vi "DatalogFile.vi"() -> ()   [LabVIEW 2019]
panel:
  in  "Boolean 2":bool
  out "Boolean":bool=TRUE
  in  "Write File":bool
  in  "Numeric 4":dbl
  in  "Numeric 3":dbl
  in  "Numeric 2":dbl
  in  "Numeric":dbl
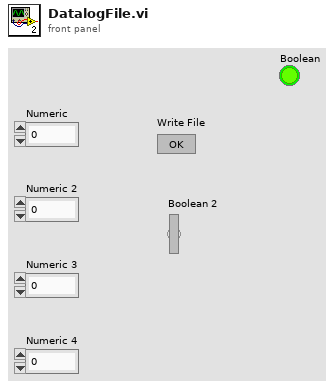
[diagram p1: front panel]
types:
  T1 = enum16{"open", "replace", "create", "open or create", "replace or create", "replace or create with confirmation"}
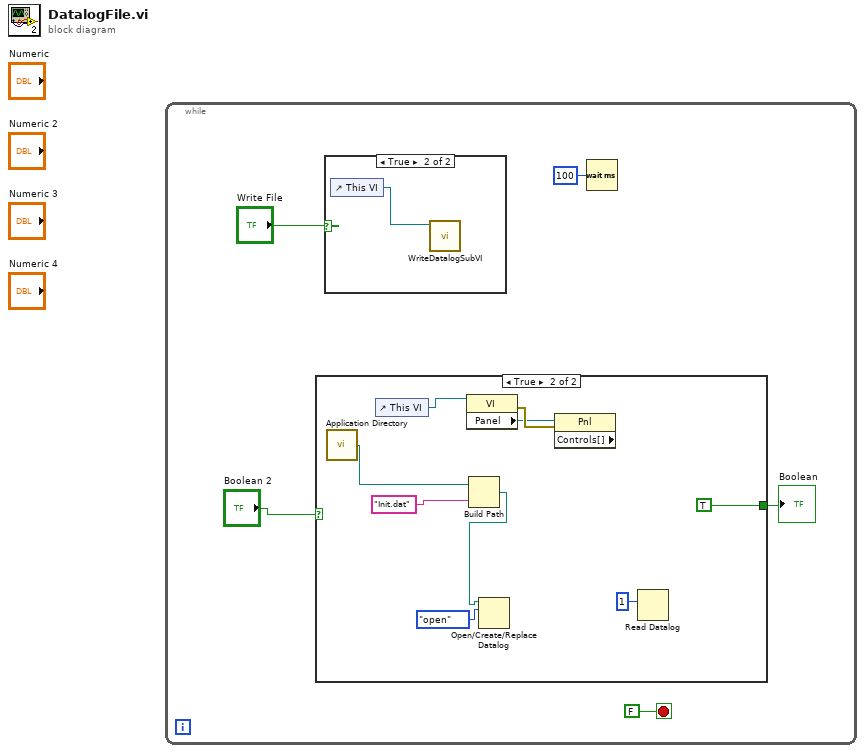
[diagram p0: block diagram]
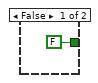
[diagram p2: hidden frame]
diagram:
  n1 = while {
    stop <- FALSE stop-if-true
    n2 = case shown="True" "Boolean 2" {
      tunnel: [FALSE TRUE] -> w2
      frame False {
      }
      frame True {
        n3 = call <vilib>:"Application Directory.vi"() -> ("Application Directory"=w14:path)
        n4 = control-ref of="This VI"() -> (w11:refnum<vi>)
        n5 = property class="VI"(reference=w11) -> (error out=w13:errorcluster, "Panel"=w12:refnum<vi>)  [unwired: 1 in, 1 out]
        n6 = Build Path(base path=w14, name or relative path="Init.dat") -> (appended path=w15:path)
        n7 = Open/Create/Replace Datalog(10:T1."open" ("operation (0:open)"), 11:w15) -> ()  [unwired: 4 in, 3 out]
        n8 = property class="Pnl" props=["Controls[]"](reference=w12, error in=w13) -> ()  [unwired: 3 out]
        n9 = Read Datalog(6:1 ("count (1)")) -> ()  [unwired: 2 in, 3 out]
      }
    }
    "Boolean" <- w2
    n10 = case shown="True" "Write File" {
      frame False {
      }
      frame True {
        n11 = control-ref of="This VI"() -> (w16:refnum<vi>)
        n12 = call "WriteDatalogSubVI.vi"("VI in"=w16) -> ()  [unwired: 11 in]
      }
    }
    n13 = Wait (ms)(milliseconds to wait=u32 100) -> ()  [unwired: 1 out]
  }
